vi "Read Config. Data.vi"(8 "error in (no error)":errorcluster, 11 "Template Action Cfg in":refnum<class "Template Action Cfg.lvclass">) -> (0 "error out":errorcluster, 2 "Config. Data":T1, 3 "Template Action Cfg out":refnum<class "Template Action Cfg.lvclass">)   [LabVIEW 2014, in "Template Action Cfg.lvclass"]
uses:
  Template Action Cfg.lvclass
  configuration data.ctl
  Template Action Cfg.lvclass/Template Action Cfg.ctl
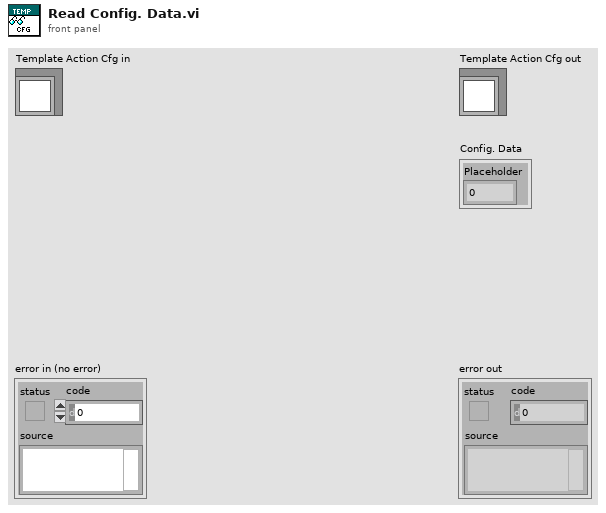
[diagram p1: front panel]
types:
  T1 = typedef "Template Action Cfg.lvclass/configuration data.ctl" = cluster{"Placeholder":dbl}
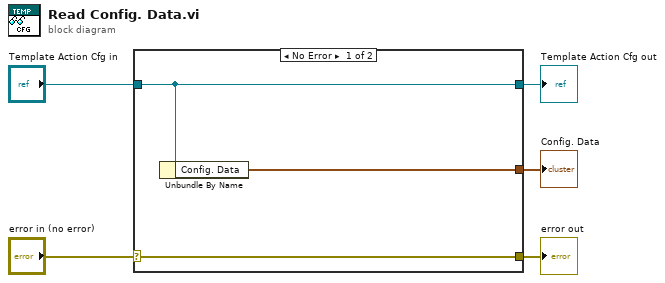
[diagram p0: block diagram]
diagram:
  n1 = case shown="No Error" "error in (no error)" {
    selector: "error in (no error)" -> [w8 w9]
    tunnel: [w8 w9] -> w4
    tunnel: [w7 w10] -> w2
    tunnel: "Template Action Cfg in" -> [w7 w10]
    tunnel: [w6 _] -> w1
    frame No Error {
      n2 = Unbundle By Name(w7) -> ("Config. Data"=w6:T1)
    }
    frame Error {
    }
  }
  "error out" <- w4
  "Template Action Cfg out" <- w2
  "Config. Data" <- w1
